vi "InitProgress.vi"() -> ()   [LabVIEW 2011]
panel:
  out "LED5":bool
  out "LED4":bool
  out "LED3":bool
  out "LED2":bool
  out "LED1":bool
  in  "EscapeRef":refnum<vi>
  in  "%Ref":refnum<vi>
  out "Processing":dbl(slide) caption="Initialisation des périphériques ..." scale=0.0..100.0
  # "Initialisation des périphériques ..."
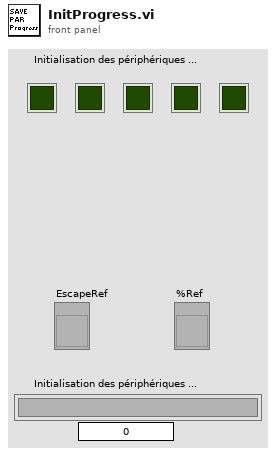
[diagram p1: front panel]
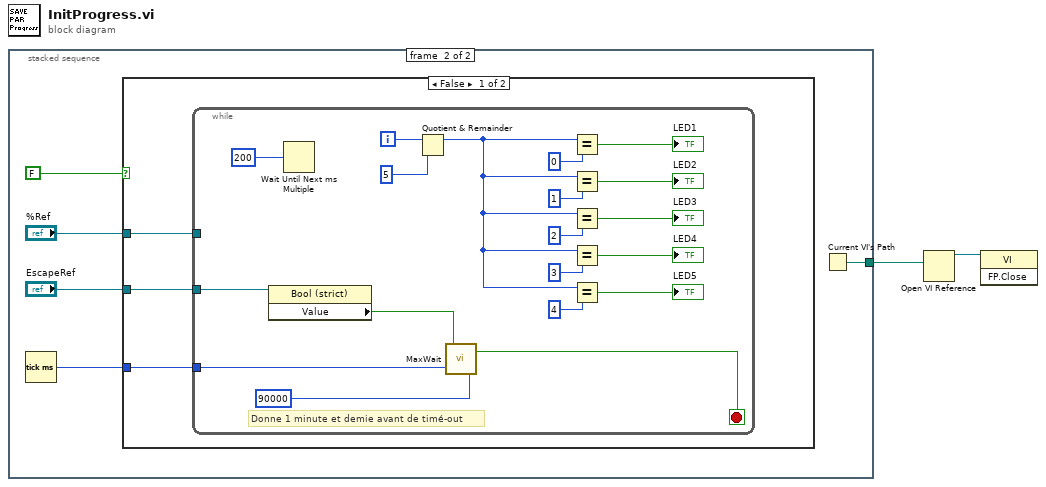
[diagram p0: block diagram]
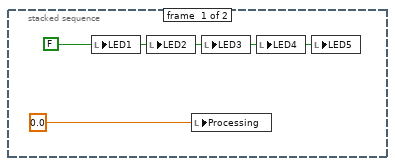
[diagram p2: hidden frame]
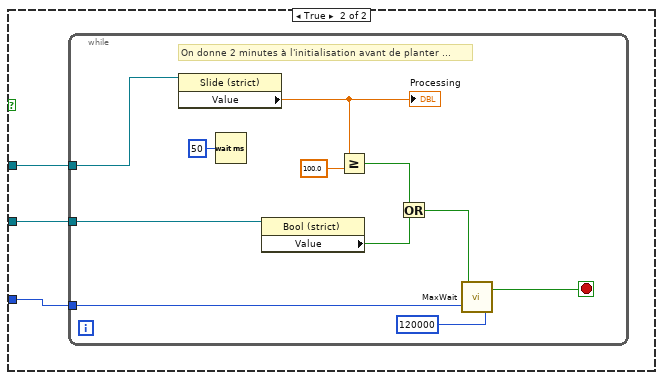
[diagram p3: hidden frame]
diagram:
  n1 = stacked-sequence {
    tunnel: [_ w5] -> w2
    frame #0 {
      w3 = FALSE ("LED1")
      n2 = local write "LED1"(w3) -> ()
      n3 = local write "LED2"(w3) -> ()
      n4 = local write "Processing"(0.0) -> ()
      n5 = local write "LED3"(w3) -> ()
      n6 = local write "LED4"(w3) -> ()
      n7 = local write "LED5"(w3) -> ()
    }
    frame #1 {
      n8 = Tick Count (ms)() -> (millisecond timer value=w7:u32)
      n9 = case shown="False" FALSE {
        tunnel: "EscapeRef" -> [w12 w34]
        tunnel: w7 -> [w11 w33]
        tunnel: "%Ref" -> [w10 w32]
        frame False {
          n10 = while {
            tunnel: w12 -> [w18]
            tunnel: w11 -> [w16]
            tunnel: w10 -> [_]
            i -> [w20]
            stop <- w15 stop-if-true
            # "Donne 1 minute et demie avant de timé-out"
            n11 = property class="Bool (strict)"(reference=w18) -> ("Value"=w13:bool)  [unwired: 1 in, 2 out]
            n12 = Wait Until Next ms Multiple(millisecond multiple=u32 200 ("milliseconds to wait")) -> ()  [unwired: 1 out]
            n13 = Quotient & Remainder(x=w20, y=5) -> (x-y*floor(x/y)=w26:i32)  [unwired: 1 out]
            n14 = call "MaxWait.vi"("WaitLimit (ms)"=u32 90000, "StartTick (from outside the node)"=w16, "Valeur entrante"=w13) -> ("break ?"=w15:bool)
            n15 = Equal?(x=w26, y=0) -> (x = y?=→"LED1":bool)
            n16 = Equal?(x=w26, y=1) -> (x = y?=→"LED2":bool)
            n17 = Equal?(x=w26, y=2) -> (x = y?=→"LED3":bool)
            n18 = Equal?(x=w26, y=3) -> (x = y?=→"LED4":bool)
            n19 = Equal?(x=w26, y=4) -> (x = y?=→"LED5":bool)
          }
        }
        frame True {
          n20 = while {
            tunnel: w33 -> [w40]
            tunnel: w34 -> [w36]
            tunnel: w32 -> [w35]
            stop <- w39 stop-if-true
            # "On donne 2 minutes à l'initialisation avant de planter ..."
            n21 = property class="Slide (strict)"(reference=w35) -> ("Value"=w44:dbl)  [unwired: 1 in, 2 out]
            "Processing" <- w44
            n22 = Wait (ms)(milliseconds to wait=u32 50) -> ()  [unwired: 1 out]
            n23 = property class="Bool (strict)"(reference=w36) -> ("Value"=w42:bool)  [unwired: 1 in, 2 out]
            n24 = Greater Or Equal?(x=w44, y=100.0) -> (x >= y?=w41:bool)
            n25 = Or(x=w41, y=w42) -> (x .or. y?=w38:bool)
            n26 = call "MaxWait.vi"("WaitLimit (ms)"=u32 120000, "StartTick (from outside the node)"=w40, "Valeur entrante"=w38) -> ("break ?"=w39:bool)
          }
        }
      }
      n27 = Current VI's Path() -> (path=w5:path)
    }
  }
  n28 = Open VI Reference(vi path=w2) -> (vi reference=w1:refnum<vi>)  [unwired: 5 in, 1 out]
  n29 = invoke class="VI" method="FP.Close"(reference=w1) -> ()  [unwired: 2 in, 3 out]
